vi "Measure Current.vi"(8 "error in":errorcluster, 11 "BKPrecision in":refnum<class "9115AT.lvclass">) -> (0 "error out":errorcluster, 2 "Current":dbl, 3 "BKPrecision out":refnum<class "9115AT.lvclass">)   [LabVIEW 2018, in "9115AT.lvlib" / "9115AT.lvclass"]
uses:
  9115AT.lvclass
  <instrlib>/BK Precision 911X Series/BK Precision 911X Series.lvlib
  builds/Power_Supply.lvlibp/Power Supply.lvclass
  C:/Users/Ron.Dexter.LUMINARTECH/Desktop/builds/Power_Supply.lvlibp/Power Supply.lvclass
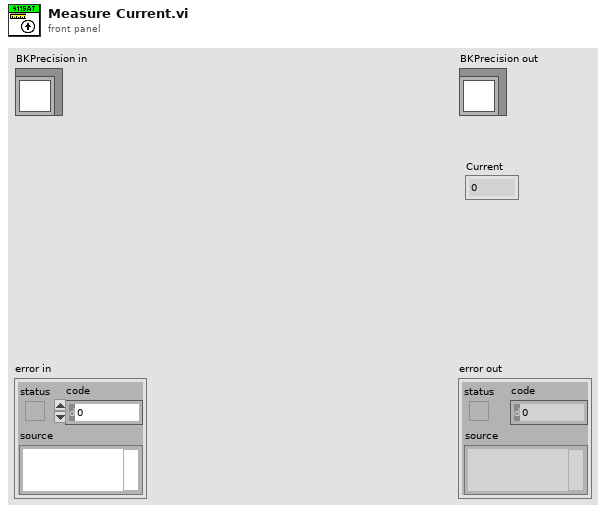
[diagram p1: front panel]
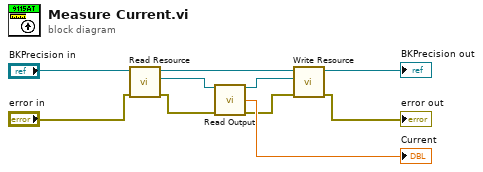
[diagram p0: block diagram]
diagram:
  n1 = call "Read Resource.vi"("error in"="error in", "Power Supply in"="BKPrecision in") -> ("error out"=w5:errorcluster, "Resource"=w6:refnum<visa-resource-name>, "Power Supply out"=w7:refnum<class "9115AT.lvclass">)  [unwired: 7 in]
  n2 = call <instrlib>:"Read Output.vi"("VISA resource name"=w6, "error in (no error)"=w5) -> ("VISA resource name out"=w3:refnum<visa-resource-name>, "Actual Current Level (A)"=→"Current":dbl, "error out"=w4:errorcluster)  [unwired: 8 in, 3 out]
  n3 = call "Write Resource.vi"("error in"=w4, "Resource"=w3, "Power Supply in"=w7) -> ("error out"=→"error out":errorcluster, "Power Supply out"=→"BKPrecision out":refnum<class "9115AT.lvclass">)  [unwired: 7 in]
